vi "GenerateWithoutData.vi"(8 "error in (no error)":errorcluster, 11 "Numeric in":refnum<class "Numeric.lvclass">) -> (0 "error out":errorcluster, 3 "Numeric out":refnum<class "Numeric.lvclass">)   [LabVIEW 2023, in "Numeric.lvclass"]
uses:
  Numeric.lvclass
  C:/Users/santharu.subramanian/Desktop/Milestone2/Sender-Receiver/Classes/Data/Data.lvclass
  Numeric.lvclass/Numeric.ctl
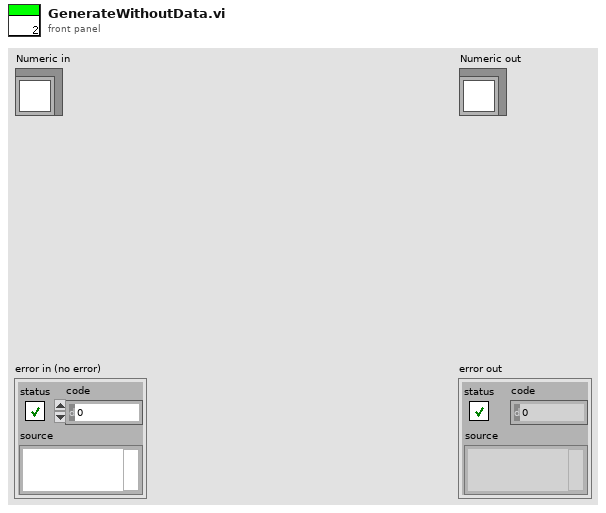
[diagram p1: front panel]
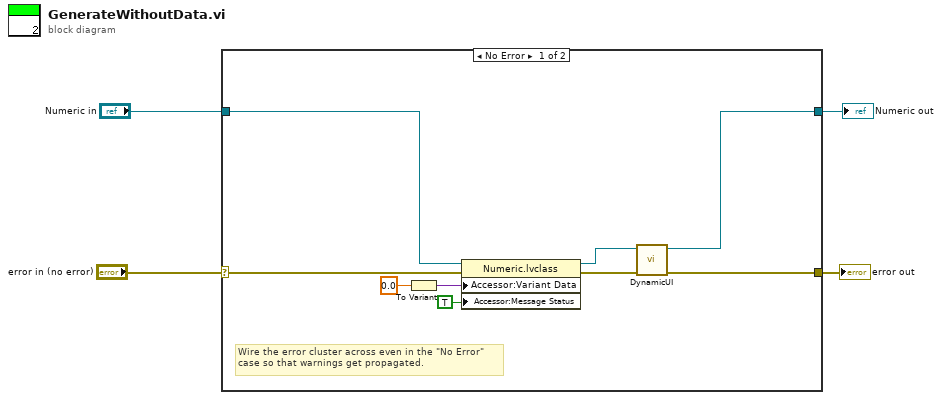
[diagram p0: block diagram]
diagram:
  n1 = case shown="No Error" "error in (no error)" {
    selector: "error in (no error)" -> [w13 w15]
    tunnel: [w6 w15] -> w3
    tunnel: [w5 w14] -> w1
    tunnel: "Numeric in" -> [w12 w14]
    frame No Error {
      # "Wire the error cluster across even in the \"No Error\"\ncase so that warnings get propagated."
      n2 = To Variant(anything=0.0) -> (Variant=w9:variant)
      n3 = property class="Numeric.lvclass"(reference=w12, error in=w13, "Accessor:Variant Data"=w9, "Accessor:Message Status"=TRUE ("Message Status")) -> (reference out=w8:refnum<class "Numeric.lvclass">, error out=w7:errorcluster)
      n4 = call "DynamicUI.vi"("error in (no error)"=w7, "Numeric in"=w8) -> ("error out"=w6:errorcluster, "Numeric out"=w5:refnum<class "Numeric.lvclass">)  [unwired: 8 in]
    }
    frame Error {
    }
  }
  "error out" <- w3
  "Numeric out" <- w1
